vi "外部窗口显示2.vi"   [LabVIEW 2018]
uses:
  <vilib>/vision/NI_Vision_Development_Module.lvlib
types:
  T1 = enum32{"Gray", "Binary", "Gradient", "Rainbow", "Temperature"}
  T2 = typedef "Image Type" = u32
  T3 = typedef "IMAQ Image.ctl" = refnum<image>
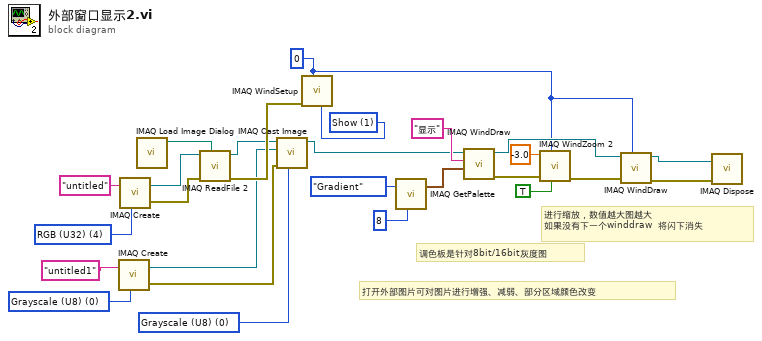
[diagram p0: block diagram]
diagram:
  w14 = T2 0 items=["Grayscale (U8)", "Grayscale (I16)", "Grayscale (SGL)", "Complex (CSG)", "RGB (U32)", "HSL (U32)", "RGB (U64)", "Grayscale (U16)"] ("Image Type")
  w15 = T2 4 items=["Grayscale (U8)", "Grayscale (I16)", "Grayscale (SGL)", "Complex (CSG)", "RGB (U32)", "HSL (U32)", "RGB (U64)", "Grayscale (U16)"] ("Image Type")
  w16 = T2 0 items=["Grayscale (U8)", "Grayscale (I16)", "Grayscale (SGL)", "Complex (CSG)", "RGB (U32)", "HSL (U32)", "RGB (U64)", "Grayscale (U16)"] ("Image Type")
  w12 = 1 items=["Hide", "Show", "No change"] ("Scrollbars (No change)")
  w1 = 0 ("Window Number (0...15)")
  # "进行缩放，数值越大图越大\n如果没有下一个winddraw  将闪下消失"
  # "打开外部图片可对图片进行增强、减弱、部分区域颜色改变"
  # "调色板是针对8bit/16bit灰度图"
  n1 = call "IMAQ Create"("Image Name"="untitled1", "Image Type"=w14) -> ("New Image"=w18:T3, "error out"=w17:errorcluster)  [unwired: 3 in]
  n2 = call "IMAQ Create"("Image Name"="untitled", "Image Type"=w15) -> ("New Image"=w24:T3, "error out"=w23:errorcluster)  [unwired: 3 in]
  n3 = call "IMAQ Load Image Dialog"() -> ("Path"=w26:path)  [unwired: 9 in, 2 out]
  n4 = call "IMAQ ReadFile 2"("File Path"=w26, "error in (no error)"=w23, "Image"=w24) -> ("error out"=w22:errorcluster, "Image Out"=w20:T3)  [unwired: 4 in, 3 out]
  n5 = call "IMAQ Cast Image"("Image Type"=w16, "error in (no error)"=w17, "Image Dst"=w18, "Image Src"=w20) -> ("Image Dst Out"=w13:T3)  [unwired: 6 in, 1 out]
  n6 = call "IMAQ WindSetup"("Scrollbars (No change)"=w12, "Window Number (0...15)"=w1, "error in (no error)"=w22) -> ()  [unwired: 8 in, 1 out]
  n7 = call "IMAQ GetPalette"("Palette Number (gray)"=T1."Gradient", "Bit Depth"=u32 8) -> ("Color Palette"=w11:cluster{"Red":u8, "Green":u8, "Blue":u8}[])  [unwired: 3 in, 1 out]
  n8 = call "IMAQ WindDraw"("Color Palette"=w11, "Title"="显示", "Image"=w13) -> ("error out"=w7:errorcluster, "Image Out (duplicate)"=w5:T3)  [unwired: 7 in]
  n9 = call "IMAQ WindZoom 2"("Get/Set Status? (Set)"=TRUE, "Window Number (0...15)"=w1, "error in (no error)"=w7, "Zoom Factor"=sgl -3.0) -> ("error out"=w4:errorcluster)  [unwired: 4 in, 3 out]
  n10 = call "IMAQ WindDraw"("Window Number (0...15)"=w1, "error in (no error)"=w4, "Image"=w5) -> ("error out"=w3:errorcluster, "Image Out (duplicate)"=w2:T3)  [unwired: 7 in]
  n11 = call "IMAQ Dispose"("Image"=w2, "error in (no error)"=w3) -> ()  [unwired: 4 in, 1 out]
